vi "Print.vi"(8 "error in (no error)":errorcluster caption="entrée d'erreur (pas d'erreur)", 11 "Class Printer_CAB en entrée":refnum<class "Class Printer_CAB.lvclass">) -> (0 "error out":errorcluster caption="sortie d'erreur", 3 "Class Printer_CAB en sortie":refnum<class "Class Printer_CAB.lvclass">)   [LabVIEW 2020, in "Library Instrument & Equipement.lvlib" / "Library Printer.lvlib" / "Class Printer_CAB.lvclass"]
uses:
  Class Printer_CAB.lvclass
  C:/Users/ngarcin/OneDrive - Altyor/Standard TB/Class/Printer/Printer (Default)/Class Printer (Default).lvclass
  Class Printer_CAB.lvclass/Class Printer_CAB.ctl
  Printer (Default)/Class Printer (Default).lvclass
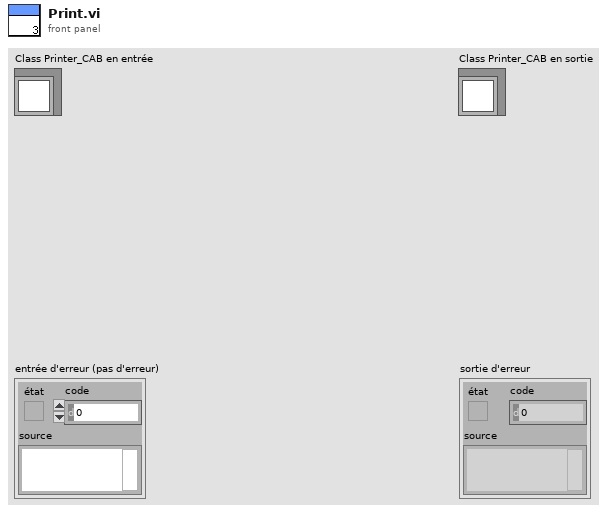
[diagram p1: front panel]
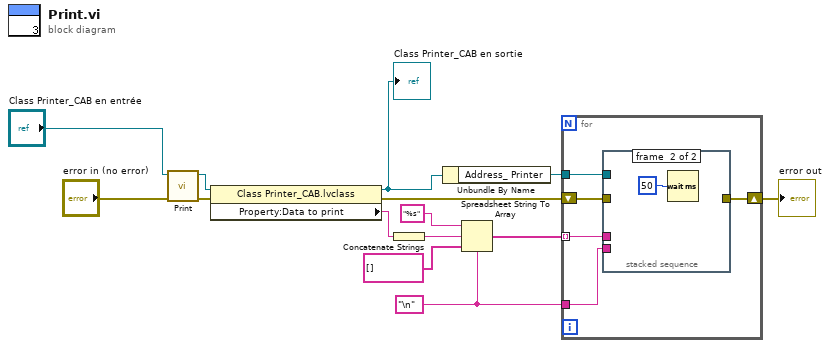
[diagram p0: block diagram]
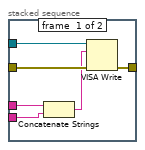
[diagram p2: hidden frame]
diagram:
  w9 = "\n" ("séparateur (Tabulation)")
  n1 = call-parent "Print.vi"("error in (no error)"="error in (no error)", "Class Printer (Default) en entrée"="Class Printer_CAB en entrée") -> ("error out"=w4:errorcluster, "Class Printer (Default) en sortie"=w3:refnum<class "Class Printer_CAB.lvclass">)  [unwired: 8 in]
  n2 = property class="Class Printer_CAB.lvclass"(reference=w3, error in=w4) -> (reference out=w1:refnum<class "Class Printer_CAB.lvclass">, error out=w2:errorcluster, "Property:Data to print"=w5:string)
  "Class Printer_CAB en sortie" <- w1
  n3 = Concatenate Strings(w5) -> (w11:string)
  n4 = Unbundle By Name(w1) -> ("Address_ Printer"=w8:refnum<visa-resource-name>)
  n5 = Spreadsheet String To Array(delimiter (Tab)=w9, format string="%s" ("chaîne de format"), spreadsheet string=w11, array type (2D Dbl)=string[] []) -> (array=w10:string[])
  n6 = for {
    shift-right: [w18] -> w7
    shift-left: w2 -> [w19]
    tunnel: w8 -> [w17]
    tunnel: w10 -> [w16] mode=indexing
    tunnel: w9 -> [w15]
    n7 = stacked-sequence {
      tunnel: w19 -> [w25 _]
      tunnel: [w24 _] -> w18
      tunnel: w17 -> [w22 _]
      tunnel: w16 -> [w21 _]
      tunnel: w15 -> [w20 _]
      frame #0 {
        n8 = Concatenate Strings(w21, w20) -> (w23:string)
        n9 = VISA Write(VISA resource name=w22, write buffer=w23, error in (no error)=w25) -> (error out=w24:errorcluster)  [unwired: 2 out]
      }
      frame #1 {
        n10 = Wait (ms)(milliseconds to wait=u32 50 ("attente (ms)")) -> ()  [unwired: 1 out]
      }
    }
  }
  "error out" <- w7
